vi "_main.vi"() -> ()   [LabVIEW 2021]
doc: "Elveflow Library\nOB1 Device\n\nExample showing how to use OB1 library with init step, calibration, and pressure regulation."
uses:
  <vilib>/ni845x/ni845x.llb/ni845xControl.ctl
  Tab_Control_PID.ctl
  Z_Regulators_type_OB1.ctl
  Z_regulator_type.ctl
  Z_Trigger_type.ctl
  Z_sensor_type.ctl
  Z_Sensor_FSD_Calib.ctl
  Z_Sensor_digit_analog.ctl
  Z_D_F_S_Resolution.ctl
  Z_Calib_type.ctl
  Z_calib_read_channel.ctl
  Z_calib_write_channel.ctl
  Z_Double_array_typedef.ctl
  OB1_Init_MK3.vi
  OB1_Init_MK4.vi
panel:
  out "Numeric":i32
  in  "error in (no error) 2":errorcluster
  in  "error in (no error)":errorcluster
  out "millisecond timer value":u32
  in  "Flow Sensor IDs":string[](array[string])
  in  "Test ID":string
  in  "operation (0:open)":T1(ring)
  in  "file path":path
  out "x-y FR":u32[](array[numeric])
  in  "stop":bool
  out "x-y Pr":u32[](array[numeric])
  in  "MK3 or MK4":bool
  in  "MK4 ressource name":refnum<visa-resource-name>
  in  "CustomS._Volt Ch4(5-25V)(Optional)":dbl
  in  "CustomS._Volt Ch3(5-25V)(Optional)":dbl
  in  "CustomS._Volt Ch2(5-25V)(Optional)":dbl
  in  "CustomS._Volt Ch1(5-25V)(Optional)":dbl
  in  "FSens_Digit_Resolution 4":T2=enum."16 bit"
  in  "FSens_Digit_Resolution 3":T2=enum."16 bit"
  in  "FSens_Digit_Resolution 2":T2=enum."16 bit"
  in  "FSens_Digit_Resolution":T2=enum."16 bit"
  out "Average Loop execution time":dbl
  in  "F.S.D Ch4 C.":T3
  in  "S.Ch4 COM":T4
  in  "S.Ch4 type":T5
  in  "S.Ch3 COM":T4
  in  "F.S.D Ch3 C.":T3
  in  "S.Ch3 type":T5
  in  "S.Ch2 COM":T4
  in  "F.S.D Ch2 C.":T3
  in  "S.Ch2 type":T5
  in  "S.Ch1 COM":T4
  in  "F.S.D Ch1 C.":T3
  in  "S.Ch1 type":T5
  out "error out":errorcluster
  in  "regulator type (MK3/MK3+)":T6
  in  "error_in":errorcluster
  in  "Tab Control":T8
  in  "Write pressure ?":bool
  in  "All Pressure\n at once":bool
  out "Graph":T9(graph)
  in  "Pressure in":dbl[](array[numeric])=[0.0, 0.0, 0.0, 0.0]
  out "Sens read":dbl[](array[numeric])
  out "Pressure read":dbl[](array[numeric])
  in  "Limits":cluster{"Max":dbl, "Min":dbl}={"Max"=300.0, "Min"=0.0}
  in  "Channel 3":cluster{"Kp":dbl, "Ti":dbl, "Td":dbl}
  in  "Channel 2":cluster{"Kp":dbl, "Ti":dbl, "Td":dbl}
  in  "Begin PID":bool
  in  "All flowrates\nat once":bool
  in  "Desired Flowrate":dbl[](array[numeric])=[0.0, 0.0, 0.0, 0.0]
  out "Sens Read":dbl[](array[numeric])
  out "Pressure Read":dbl[](array[numeric])
  out "Graph":T9(graph)
  in  "Channel 1":cluster{"Kp":dbl, "Ti":dbl, "Td":dbl}
  in  "reinitialize? (F)":bool
  out "Get Trigger Input":T10
  in  "Set Trigger Output":T10
  in  "Calibration":T11(tab)
  out "Progress bar":u8(slide) scale=0.0..100.0
  in  "Path":path
  in  "MK3/MK3+ ressource name":T12
  # "Pressure Controller Code"
  # "CALIB (choose the calib\nbefore the VI run)"
  # "milliseconds"
  # "INIT (Configure it before the VI run)"
  # "USE (main acquisition loop)"
  # "MK3/MK3+"
  # "MK4"
  # "Flow Sensor\nDigital \nCalibration"
  # "Sensor\nAnalog/\nDigital"
  # "Flow Sensor\nDigital \nResolution"
  # "Custom Sensor Voltage (only valid for OB1 bought in 2020 and after)"
  # "Sensor TYPE"
  # "Copy and paste the directory of the location you want to save the data, followed by \\[pick a filename]"
  # "Channel 1"
  # "Channel 2"
  # "Channel 3"
  # "PID Gains"
  # "this tab active = Use default calibration"
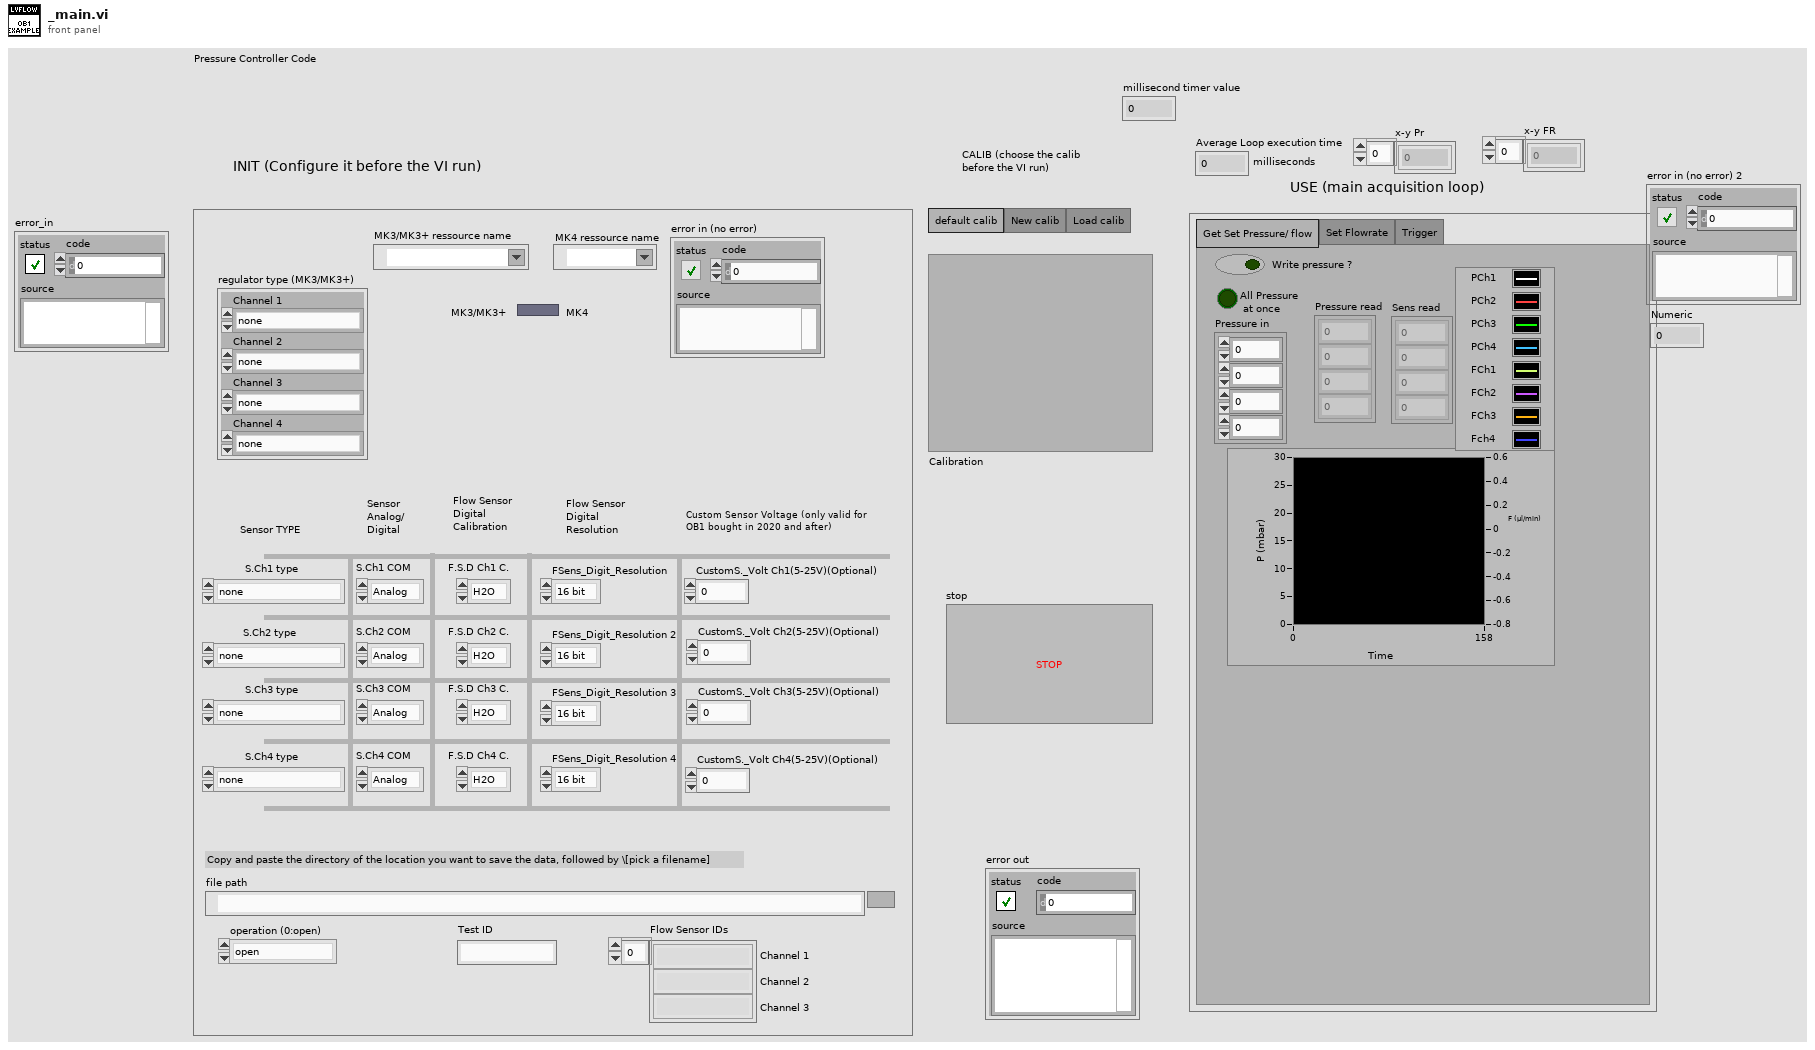
[diagram p1: front panel]
types:
  T1 = enum16{"open", "open or create", "create or replace", "create", "open (read-only)"}
  T2 = typedef "Z_D_F_S_Resolution.ctl" = enum16{"9 bit", "10 bit", "11 bit", "12 bit", "13 bit", "14 bit", "15 bit", "16 bit"}
  T3 = typedef "Z_Sensor_FSD_Calib.ctl" = enum16{"H2O", "IPA"}
  T4 = typedef "Z_Sensor_digit_analog.ctl" = enum16{"Analog", "Digital"}
  T5 = typedef "Z_sensor_type.ctl" = enum16{"none", "Flow_1_5_muL_min", "Flow_7_muL_min", "Flow_50_muL_min", "Flow_80_muL_min", "Flow_1000_muL_min", "Flow_5000_muL_min", "Press_70_mbar", "Press_340_mbar", "Press_1_bar", "Press_2_bar", "Press_7_bar", "Press_16_bar", "Level", "Custom"}
  T6 = typedef "Z_Regulators_type_OB1.ctl" = cluster{"Channel 1":T7, "Channel 2":T7, "Channel 3":T7, "Channel 4":T7}
  T7 = typedef "Z_regulator_type.ctl" = enum16{"none", "0_200_mbar", "0_2000_mbar", "0_8000_mbar", "m1000_1000_mbar", "m1000_6000_mbar"}
  T8 = typedef "Tab_Control_PID.ctl" = enum32{"Get Set Pressure/ flow", "Set Flowrate", "Trigger"}
  T9 = cluster{"Pressure array[0]":dbl, "Pressure array[1]":dbl, "Pressure array[2]":dbl, "Pressure array[3]":dbl, "Pressure array[4]":dbl, "Pressure array[5]":dbl, "Pressure array[6]":dbl, "Pressure array[7]":dbl, "Pressure array[8]":dbl}
  T10 = typedef "Z_Trigger_type.ctl" = enum16{"Low", "High"}
  T11 = enum32{"default calib", "New calib", "Load calib"}
  T12 = typedef "ni845xControl.ctl" = refnum<k21>
  T13 = cluster{"Meas Pressure":dbl[], "Meas Flowrate":dbl[], "Current Time":dbl, "Start Time":dbl, "Ref Pressure":dbl[], "Ref Flowrate":dbl[], "Flowrate Limits":cluster{"Max":dbl, "Min":dbl}, "Chan 1 Gains":cluster{"Kp":dbl, "Ti":dbl, "Td":dbl}, "Chan 2 Gains":cluster{"Kp":dbl, "Ti":dbl, "Td":dbl}, "Chan 3 Gains":cluster{"Kp":dbl, "Ti":dbl, "Td":dbl}}
  T14 = typedef "Z_OB1_type.ctl" = cluster{"DevName out":string, "OB1 type":T15, "regulator type":cluster{"channel 1":T7, "channel 2":T7, "channel 3":T7, "channel 4":T7}, "OB1_Sens_type":T16, "SPI configs":T18, "Row Reg and Sens data MK3":u16[], "Calibration Regulators":cluster{"Calibrated":bool, "Offset":dbl, "Slope":dbl, "ID regulator":string}[], "Row Reg and Sens data MK4":string}
  T15 = typedef "Z_OB1_Version.ctl" = enum16{"MK3-V1", "MK3-V2", "MK3-V3", "MK4_V1"}
  T16 = typedef "Z_Sensors_type_OB1.ctl" = cluster{"Ch1":T17, "Ch2":T17, "Ch3":T17, "Ch4":T17}
  T17 = typedef "Z_OB1_sensor_type.ctl" = cluster{"Sensor_type":T5, "Digital/Analog":T4, "Sensirion_Digit_Calib":T3, "Sensirion_Calib_factor":dbl, "Sensirion_Digit_Resolution":T2, "Custom_Sensor_Voltage":dbl}
  T18 = typedef "Z_OB1_SPI_Cfg.ctl" = cluster{"Get S_analog ang R":T19}
  T19 = typedef "ni845xSpiScriptControl.ctl" = refnum<k20>
  T20 = typedef "Z_Calib_type.ctl" = cluster{"default calibration ?":bool, "calib reading ":T21[], "calib write all channel":T22[]}
  T21 = typedef "Z_calib_read_channel.ctl" = cluster{"offset":dbl, "slope ":dbl}
  T22 = typedef "Z_calib_write_channel.ctl" = cluster{"target_pressures":T23, "read_pressures":T23}
  T23 = typedef "Z_Double_array_typedef.ctl" = dbl[]
  T24 = cluster{"[0]":dbl, "[1]":dbl, "[2]":dbl, "[3]":dbl, "[4]":dbl, "[5]":dbl, "[6]":dbl, "[7]":dbl, "[8]":dbl}
  T25 = cluster{dbl[][], dbl[][], dbl[][], dbl[][], dbl[][]}
  T26 = cluster{"Chan 3 Gains":cluster{"Kp":dbl, "Ti":dbl, "Td":dbl}}[]
  T27 = cluster{"Meas Flowrate[0]":dbl, "Meas Flowrate[1]":dbl, "Meas Flowrate[2]":dbl, "Meas Flowrate[3]":dbl, "Meas Flowrate[4]":dbl, "Meas Flowrate[5]":dbl, "Meas Flowrate[6]":dbl, "Meas Flowrate[7]":dbl, "Meas Flowrate[8]":dbl}
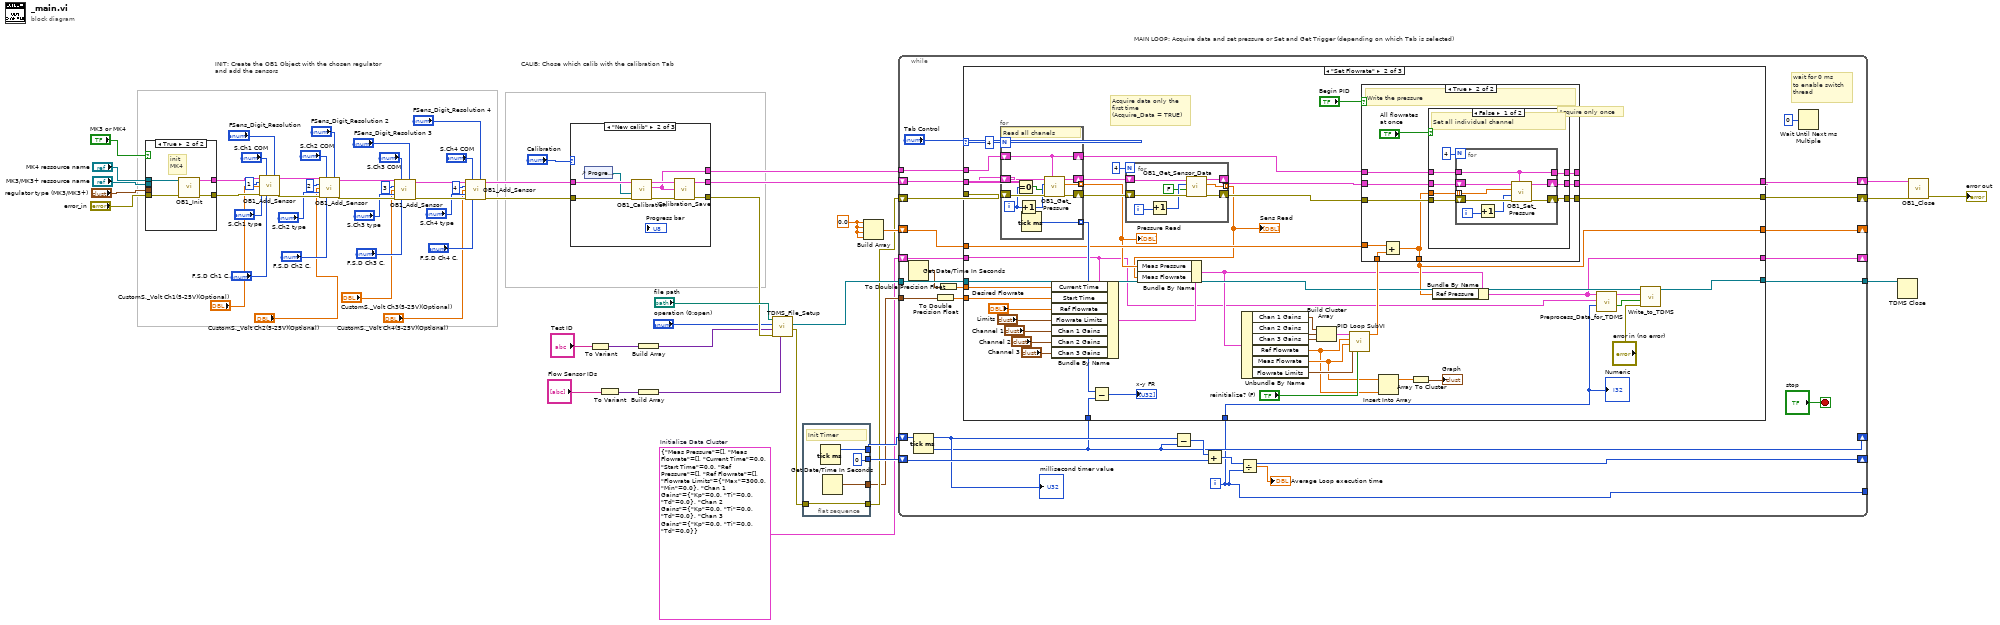
[diagram p0: block diagram]
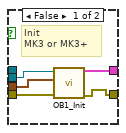
[diagram p2: hidden frame]
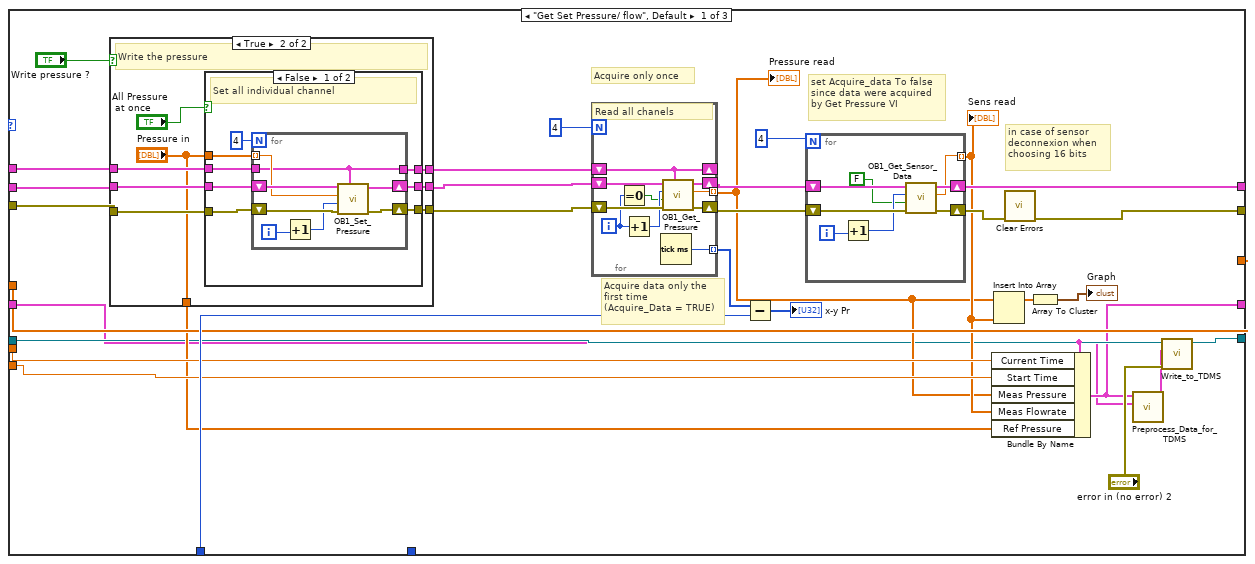
[diagram p3: hidden frame]
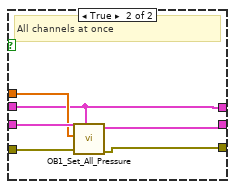
[diagram p5: hidden frame]
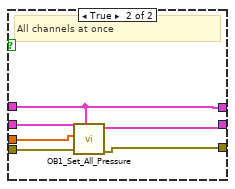
[diagram p7: hidden frame]
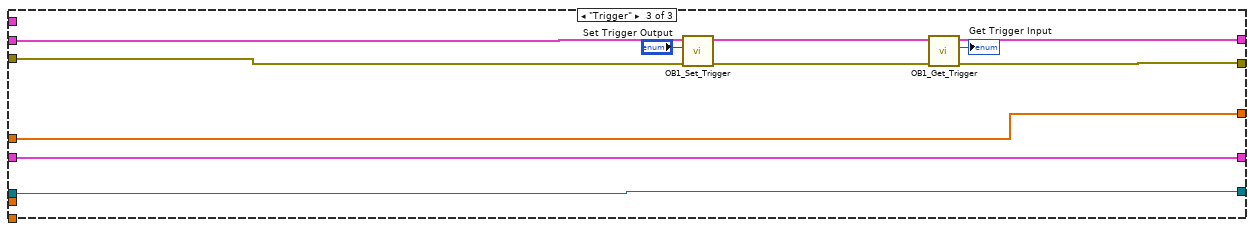
[diagram p8: hidden frame]
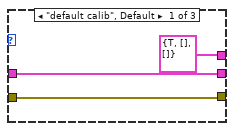
[diagram p9: hidden frame]
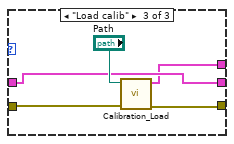
[diagram p10: hidden frame]
diagram:
  w1 = T13 {"Meas Pressure"=[], "Meas Flowrate"=[], "Current Time"=0.0, "Start Time"=0.0, "Ref Pressure"=[], "Ref Flowrate"=[], "Flowrate Limits"={"Max"=300.0, "Min"=0.0}, "Chan 1 Gains"={"Kp"=0.0, "Ti"=0.0, "Td"=0.0}, "Chan 2 Gains"={"Kp"=0.0, "Ti"=0.0, "Td"=0.0}, "Chan 3 Gains"={"Kp"=0.0, "Ti"=0.0, "Td"=0.0}}  # Initialize Data Cluster
  w17 = 0.0 ("element")
  # "MAIN LOOP: Acquire data and set pressure or Set and Get Trigger (depending on which Tab is selected)"
  # "CALIB: Chose which calib with the calibration Tab"
  # "INIT: Create the OB1 Object with the chosen regulator\nand add the sensors"
  n1 = case shown="True" "MK3 or MK4" {
    tunnel: "error_in" -> [w67 w73]
    tunnel: [w65 w72] -> w60
    tunnel: [w66 w71] -> w59
    tunnel: "MK4 ressource name" -> [_ w70]
    tunnel: "MK3/MK3+ ressource name" -> [w69 _]
    tunnel: "regulator type (MK3/MK3+)" -> [w68 _]
    frame False {
      # "Init\nMK3 or MK3+"
      n2 = call-poly "OB1_Init.vi"("error in"=w67, "regulator type"=w68, "device reference"=w69) -> ("error_out"=w66:errorcluster, "OB1 cluster (out)"=w65:T14)  [unwired: 7 in]
    }
    frame True {
      # "init\nMK4"
      n3 = call-poly "OB1_Init.vi"("error in"=w73, "VISA resource name"=w70) -> ("error_out"=w71:errorcluster, "OB1 cluster (out)"=w72:T14)  [unwired: 8 in]
    }
  }
  n4 = call "OB1_Add_Sensor.vi"("OB1 cluster (in)"=w60, "Digital/Analog"="S.Ch1 COM", "FSens_Digit_Resolution"="FSens_Digit_Resolution", "Channel_1_to_4"=1 ("Channel (1-4)"), "Custom_Sensor_Voltage in (5-25V) (Optional)"="CustomS._Volt Ch1(5-25V)(Optional)", "Sensor type"="S.Ch1 type", "error in"=w59, "FSens_Digit_Calib"="F.S.D Ch1 C.") -> ("OB1 cluster (out)"=w54:T14, "error out"=w53:errorcluster)  [unwired: 6 in]
  n5 = call "OB1_Add_Sensor.vi"("OB1 cluster (in)"=w54, "Digital/Analog"="S.Ch2 COM", "FSens_Digit_Resolution"="FSens_Digit_Resolution 2", "Channel_1_to_4"=2 ("Channel (1-4)"), "Custom_Sensor_Voltage in (5-25V) (Optional)"="CustomS._Volt Ch2(5-25V)(Optional)", "Sensor type"="S.Ch2 type", "error in"=w53, "FSens_Digit_Calib"="F.S.D Ch2 C.") -> ("OB1 cluster (out)"=w48:T14, "error out"=w43:errorcluster)  [unwired: 6 in]
  n6 = call "OB1_Add_Sensor.vi"("OB1 cluster (in)"=w48, "Digital/Analog"="S.Ch3 COM", "FSens_Digit_Resolution"="FSens_Digit_Resolution 3", "Channel_1_to_4"=3 ("Channel (1-4)"), "Custom_Sensor_Voltage in (5-25V) (Optional)"="CustomS._Volt Ch3(5-25V)(Optional)", "Sensor type"="S.Ch3 type", "error in"=w43, "FSens_Digit_Calib"="F.S.D Ch3 C.") -> ("OB1 cluster (out)"=w47:T14, "error out"=w44:errorcluster)  [unwired: 6 in]
  n7 = call "OB1_Add_Sensor.vi"("OB1 cluster (in)"=w47, "Digital/Analog"="S.Ch4 COM", "FSens_Digit_Resolution"="FSens_Digit_Resolution 4", "Channel_1_to_4"=4, "Custom_Sensor_Voltage in (5-25V) (Optional)"="CustomS._Volt Ch4(5-25V)(Optional)", "Sensor type"="S.Ch4 type", "error in"=w44, "FSens_Digit_Calib"="F.S.D Ch4 C.") -> ("OB1 cluster (out)"=w46:T14, "error out"=w45:errorcluster)  [unwired: 6 in]
  n8 = case shown="\"New calib\"" "Calibration" {
    tunnel: w45 -> [w75 w83 w87]
    tunnel: w46 -> [w76 w82 w86]
    tunnel: [w76 w81 w86] -> w26
    tunnel: [w75 w80 w85] -> w14
    tunnel: [T20 {"default calibration ?"=TRUE, "calib reading "=[], "calib write all channel"=[]} ("Calibration") w79 w84] -> w28
    frame "default calib", Default {
    }
    frame "New calib" {
      n9 = control-ref of="Progress bar"() -> (w77:refnum<vi>)
      n10 = call "OB1_Calibration.vi"("error in"=w83, "Ref num to Slide"=w77, "OB1 cluster (in)"=w82) -> ("error out"=w78:errorcluster, "Calibration"=w79:T20, "OB1 cluster (out)"=w81:T14)  [unwired: 6 in]
      n11 = call "Calibration_Save.vi"("error in"=w78, "Calibration"=w79) -> ("error out"=w80:errorcluster)  [unwired: 9 in]
    }
    frame "Load calib" {
      n12 = call "Calibration_Load.vi"("error in"=w87, "Path"="Path") -> ("error out"=w85:errorcluster, "Calibration"=w84:T20)  [unwired: 7 in, 1 out]
    }
  }
  n13 = To Variant(anything="Test ID") -> (Variant=w9:variant)
  n14 = To Variant(anything="Flow Sensor IDs") -> (Variant=w6:variant)
  n15 = Build Array(w6) -> (w5:variant[])
  n16 = Build Array(w9) -> (w8:variant[])
  n17 = call "TDMS_File_Setup.vi"("Sensor IDs"=w5, "error in (no error)"=w14, "TestID"=w8, "operation (0:open)"="operation (0:open)", "file path"="file path") -> ("error out"=w4:errorcluster, "tdms file out"=w12:refnum<k34>)  [unwired: 5 in]
  n18 = flat-sequence {
    tunnel: w4 -> [w90]
    tunnel: [w92] -> w34
    tunnel: [u64 0] -> w33
    tunnel: [w90] -> w3
    tunnel: [w89] -> w2
    frame #0 {
      # "Init Timer"
      n19 = Tick Count (ms)() -> (millisecond timer value=w92:u32)
      n20 = Get Date/Time In Seconds() -> (seconds since 1Jan1904=w89:timestamp)
    }
  }
  n21 = Build Array(w17, w17, w17, w17) -> (w16:dbl[])
  n22 = while {
    shift-right: [w113] -> w64
    shift-left: w26 -> [w117]
    tunnel: w28 -> [w115]
    shift-right: [w105] -> _
    shift-left: w34 -> [w108]
    shift-right: [w107] -> w27
    shift-left: w3 -> [w116]
    tunnel: [w93] -> _
    shift-right: [w111] -> _
    shift-left: w33 -> [w110]
    shift-right: [w103] -> _
    shift-left: w16 -> [w104]
    tunnel: w12 -> [w101]
    tunnel: [w100] -> w11
    tunnel: w2 -> [w99]
    shift-right: [w94] -> _
    shift-left: w1 -> [w97]
    i -> [w93]
    stop <- "stop" stop-if-true
    # "wait for 0 ms\nto enable switch \nthread"
    n23 = Get Date/Time In Seconds() -> (seconds since 1Jan1904=w96:timestamp)
    n24 = Tick Count (ms)() -> (millisecond timer value=w105:u32)
    n25 = To Double Precision Float(number=w99) -> (double precision float=w98:dbl)
    n26 = To Double Precision Float(number=w96) -> (double precision float=w95:dbl)
    n27 = case shown="\"Set Flowrate\"" "Tab Control" {
      tunnel: w117 -> [w140 w236 w310]
      tunnel: w116 -> [w139 w234 w309]
      tunnel: w115 -> [w141 w239 _]
      tunnel: [w135 w237 w308] -> w113
      tunnel: [w134 w226 w307] -> w107
      tunnel: w105 -> [w131 w243 _]
      tunnel: w104 -> [w129 w230 w304]
      tunnel: [w129 w213 w304] -> w103
      tunnel: w101 -> [w122 w224 w303]
      tunnel: [w121 w223 w303] -> w100
      tunnel: w98 -> [w127 w221 _]
      tunnel: w97 -> [w118 w202 w302]
      tunnel: w95 -> [w128 w204 _]
      tunnel: [w119 w203 w302] -> w94
      tunnel: w93 -> [_ w200 _]
      frame "Get Set Pressure/ flow", Default {
        # "in case of sensor\ndeconnexion when\nchoosing 16 bits"
        # "set Acquire_data To false \nsince data were acquired \nby Get Pressure VI"
        # "Acquire data only the \nfirst time \n(Acquire_Data = TRUE)"
        # "Acquire only once"
        n28 = case shown="True" "Write pressure ?" {
          tunnel: w140 -> [w150 w159]
          tunnel: w139 -> [w149 w158]
          tunnel: w141 -> [w151 w157]
          tunnel: [w149 w155] -> w136
          tunnel: [w150 w154] -> w137
          tunnel: [w151 w153] -> w138
          tunnel: [_ "Pressure in"] -> w126
          frame False {
            # "Read the pressure only"
          }
          frame True {
            # "Write the pressure"
            n29 = case shown="False" "All Pressure\n at once" {
              tunnel: [w167 w178] -> w154
              tunnel: [w166 w177] -> w155
              tunnel: w159 -> [w165 w181]
              tunnel: w158 -> [w164 w179]
              tunnel: w157 -> [w163 w176]
              tunnel: [w162 w176] -> w153
              tunnel: "Pressure in" -> [w161 w180]
              frame False {
                # "Set all individual channel"
                n30 = for {
                  N: 4 -> [_]
                  shift-right: [w173] -> w167
                  shift-left: w165 -> [w174]
                  shift-right: [w172] -> w166
                  shift-left: w164 -> [w175]
                  tunnel: w161 -> [w171] mode=indexing
                  tunnel: w163 -> [w168]
                  tunnel: [w168] -> w162
                  i -> [w170]
                  n31 = Increment(x=w170) -> (x+1=w169:i32)
                  n32 = call "OB1_Set_Pressure.vi"("calib cluster"=w168, "error in"=w175, "Channel_1_to_4"=w169, "Pressure"=w171, "OB1 cluster (in)"=w174) -> ("error out"=w172:errorcluster, "OB1 cluster (out)"=w173:T14)  [unwired: 5 in]
                }
              }
              frame True {
                # "All channels at once"
                n33 = call "OB1_Set_All_Pressure.vi"("calib cluster"=w176, "error in"=w179, "Pressure Array"=w180, "OB1 cluster (in)"=w181) -> ("error out"=w177:errorcluster, "OB1 cluster (out)"=w178:T14)  [unwired: 6 in]
              }
            }
          }
        }
        n34 = for {
          N: 4 -> [_]
          tunnel: [w197] -> w124 mode=indexing
          shift-right: [w196] -> w147
          shift-left: w137 -> [w199]
          shift-right: [w191] -> w146
          shift-left: w136 -> [w198]
          shift-right: [w194] -> _
          shift-left: w138 -> [w194]
          tunnel: [w190] -> w132 mode=indexing
          i -> [w193]
          # "Read all chanels"
          n35 = Equal To 0?(x=w193) -> (x = 0?=w192:bool)
          n36 = Increment(x=w193) -> (x+1=w195:i32)
          n37 = Tick Count (ms)() -> (millisecond timer value=w190:u32)
          n38 = call "OB1_Get_Pressure.vi"("Calibration"=w194, "error in"=w198, "Acquire_Data"=w192, "Channel_1_to_4"=w195, "OB1 cluster (in)"=w199) -> ("error in"=w191:errorcluster, "Pressure"=w197:dbl, "OB1 cluster (out)"=w196:T14)  [unwired: 4 in]
        }
        "Pressure read" <- w124
        n39 = Subtract(x=w132, y=w131) -> (x-y=→"x-y Pr":u32[])
        n40 = for {
          N: 4 -> [_]
          shift-right: [w185] -> w135
          shift-left: w147 -> [w188]
          shift-right: [w182] -> w143
          shift-left: w146 -> [w187]
          tunnel: [w184] -> w125 mode=indexing
          i -> [w189]
          n41 = Increment(x=w189) -> (x+1=w186:i32)
          n42 = call "OB1_Get_Sensor_Data.vi"("error in"=w187, "Acquire_Data"=FALSE, "Channel_1_to_4"=w186, "OB1 cluster (in)"=w188) -> ("error out"=w182:errorcluster, "Sens_Data"=w184:dbl, "OB1 cluster (out)"=w185:T14)  [unwired: 5 in]
        }
        "Sens read" <- w125
        n43 = Bundle By Name(cluster=w118, "Current Time"=w128, "Start Time"=w127, "Meas Pressure"=w124, "Meas Flowrate"=w125, "Ref Pressure"=w126) -> (w119:T13)
        n44 = Insert Into Array(array=w124, new element=w125) -> (w133:dbl[])  [unwired: 1 in]
        n45 = call <vilib>:"Clear Errors.vi"("error in (no error)"=w143) -> ("error out"=w134:errorcluster)  [unwired: 5 in, 1 out]
        n46 = Array To Cluster(array=w133) -> (cluster=→"Graph":T24)
        n47 = call "Preprocess_Data_for_TDMS.vi"("Previous Cluster"=w118, "Current Cluster"=w119) -> ("output cluster"=w120:T25)  [unwired: 7 in, 2 out]
        n48 = call "Write_to_TDMS.vi"("error in (no error)"="error in (no error) 2", "output cluster"=w120, "Refnum in"=w122) -> ("Refnum out"=w121:refnum<k34>)  [unwired: 8 in]
      }
      frame "Set Flowrate" {
        # "Acquire data only the \nfirst time \n(Acquire_Data = TRUE)"
        # "Acquire only once"
        n49 = for {
          N: 4 -> [_]
          tunnel: [w255] -> w209 mode=indexing
          shift-right: [w254] -> w235
          shift-left: w236 -> [w257]
          shift-right: [w249] -> w233
          shift-left: w234 -> [w256]
          shift-right: [w252] -> w238
          shift-left: w239 -> [w252]
          tunnel: [w248] -> w232 mode=indexing
          i -> [w251]
          # "Read all chanels"
          n50 = Equal To 0?(x=w251) -> (x = 0?=w250:bool)
          n51 = Increment(x=w251) -> (x+1=w253:i32)
          n52 = Tick Count (ms)() -> (millisecond timer value=w248:u32)
          n53 = call "OB1_Get_Pressure.vi"("Calibration"=w252, "error in"=w256, "Acquire_Data"=w250, "Channel_1_to_4"=w253, "OB1 cluster (in)"=w257) -> ("error in"=w249:errorcluster, "Pressure"=w255:dbl, "OB1 cluster (out)"=w254:T14)  [unwired: 4 in]
        }
        "Pressure Read" <- w209
        n54 = Bundle By Name(cluster=w202, "Current Time"=w204, "Start Time"=w221, "Ref Flowrate"="Desired Flowrate", "Flowrate Limits"="Limits", "Chan 1 Gains"="Channel 1", "Chan 2 Gains"="Channel 2", "Chan 3 Gains"="Channel 3") -> (w210:T13)
        n55 = Subtract(x=w232, y=w243) -> (x-y=→"x-y FR":u32[])
        n56 = for {
          N: 4 -> [_]
          shift-right: [w297] -> w245
          shift-left: w235 -> [w300]
          shift-right: [w294] -> w227
          shift-left: w233 -> [w299]
          tunnel: [w296] -> w208 mode=indexing
          i -> [w301]
          n57 = Increment(x=w301) -> (x+1=w298:i32)
          n58 = call "OB1_Get_Sensor_Data.vi"("error in"=w299, "Acquire_Data"=FALSE, "Channel_1_to_4"=w298, "OB1 cluster (in)"=w300) -> ("error out"=w294:errorcluster, "Sens_Data"=w296:dbl, "OB1 cluster (out)"=w297:T14)  [unwired: 5 in]
        }
        "Sens Read" <- w208
        n59 = Bundle By Name(cluster=w210, "Meas Pressure"=w209, "Meas Flowrate"=w208) -> (w207:T13)
        n60 = Unbundle By Name(w207) -> ("Chan 1 Gains"=w217:cluster{"Kp":dbl, "Ti":dbl, "Td":dbl}, "Chan 2 Gains"=w216:cluster{"Kp":dbl, "Ti":dbl, "Td":dbl}, "Chan 3 Gains"=w215:cluster{"Kp":dbl, "Ti":dbl, "Td":dbl}, "Ref Flowrate"=w205:dbl[], "Meas Flowrate"=w206:dbl[], "Flowrate Limits"=w214:cluster{"Max":dbl, "Min":dbl})
        n61 = Build Cluster Array(w217, w216, w215) -> (w228:T26)
        n62 = call "PID Loop SubVI.vi"("reinitialize? (F)"="reinitialize? (F)", "Output Limits"=w214, "Measured Flowrate"=w206, "Desired Flowrate"=w205, "Gains"=w228) -> ("Array out"=w231:dbl[])  [unwired: 6 in]
        n63 = case shown="True" "Begin PID" {
          tunnel: w245 -> [w260 w271]
          tunnel: w227 -> [w259 w270]
          tunnel: w238 -> [w261 w269]
          tunnel: [w259 w268] -> w226
          tunnel: [w260 w267] -> w237
          tunnel: [w261 w266] -> _
          tunnel: w231 -> [_ w262]
          tunnel: w230 -> [w258 w263]
          tunnel: [w258 w264] -> w213
          frame False {
            # "Read the pressure only"
          }
          frame True {
            # "Write the pressure"
            n64 = Add(x=w263, y=w262) -> (x+y=w264:dbl[])
            n65 = case shown="False" "All flowrates\nat once" {
              tunnel: [w279 w290] -> w267
              tunnel: [w278 w289] -> w268
              tunnel: w271 -> [w277 w293]
              tunnel: w270 -> [w276 w291]
              tunnel: w269 -> [w275 w288]
              tunnel: [w274 w288] -> w266
              tunnel: w264 -> [w273 w292]
              frame False {
                # "Set all individual channel"
                n66 = for {
                  N: 4 -> [_]
                  shift-right: [w285] -> w279
                  shift-left: w277 -> [w286]
                  shift-right: [w284] -> w278
                  shift-left: w276 -> [w287]
                  tunnel: w273 -> [w283] mode=indexing
                  tunnel: w275 -> [w280]
                  tunnel: [w280] -> w274
                  i -> [w282]
                  n67 = Increment(x=w282) -> (x+1=w281:i32)
                  n68 = call "OB1_Set_Pressure.vi"("calib cluster"=w280, "error in"=w287, "Channel_1_to_4"=w281, "Pressure"=w283, "OB1 cluster (in)"=w286) -> ("error out"=w284:errorcluster, "OB1 cluster (out)"=w285:T14)  [unwired: 5 in]
                }
              }
              frame True {
                # "All channels at once"
                n69 = call "OB1_Set_All_Pressure.vi"("calib cluster"=w288, "error in"=w291, "Pressure Array"=w292, "OB1 cluster (in)"=w293) -> ("error out"=w289:errorcluster, "OB1 cluster (out)"=w290:T14)  [unwired: 6 in]
              }
            }
          }
        }
        n70 = Insert Into Array(array=w206, new element=w205) -> (w241:dbl[])  [unwired: 1 in]
        n71 = Array To Cluster(array=w241) -> (cluster=→"Graph":T27)
        n72 = Bundle By Name(cluster=w207, "Ref Pressure"=w213) -> (w203:T13)
        n73 = call "Preprocess_Data_for_TDMS.vi"("Super Loop Index"=w200, "Previous Cluster"=w202, "Current Cluster"=w203) -> ("appended array"=w201:bool[], "output cluster"=w225:T25)  [unwired: 6 in, 1 out]
        n74 = call "Write_to_TDMS.vi"("error in (no error)"="error in (no error)", "Array"=w201, "output cluster"=w225, "Refnum in"=w224) -> ("Refnum out"=w223:refnum<k34>)  [unwired: 7 in]
        "Numeric" <- w200
      }
      frame "Trigger" {
        n75 = call "OB1_Set_Trigger.vi"("error in (no error)"=w309, "Trigger"="Set Trigger Output", "OB1 cluster (in)"=w310) -> ("error out"=w311:errorcluster, "OB1 cluster (out)"=w312:T14)  [unwired: 7 in]
        n76 = call "OB1_Get_Trigger.vi"("error in"=w311, "OB1 cluster (in)"=w312) -> ("error out"=w307:errorcluster, "Trigger_out"=→"Get Trigger Input":T10, "OB1 cluster (out)"=w308:T14)  [unwired: 7 in]
      }
    }
    n77 = Subtract(x=w105, y=w108) -> (x-y=w112:u32)
    n78 = Add(x=w112, y=w110) -> (x+y=w111:u64)
    n79 = Divide(x=w111, y=w93) -> (x/y=→"Average Loop execution time":dbl)
    n80 = Wait Until Next ms Multiple(millisecond multiple=u32 0) -> ()  [unwired: 1 out]
    "millisecond timer value" <- w108
  }
  n81 = TDMS Close(11:w11) -> ()  [unwired: 1 in, 2 out]
  n82 = call "OB1_Close.vi"("error in"=w27, "OB1 cluster (in)"=w64) -> ("error out"=→"error out":errorcluster)  [unwired: 9 in]
